vi "Set Defaults.vi"(8 "error in":errorcluster, 11 "VISA resource name":refnum<visa-resource-name>) -> (0 "error out":errorcluster, 3 "VISA resource name out":refnum<visa-resource-name>)   [LabVIEW 2019, in "Acopian.lvlib" / "Acopian.lvclass"]
uses:
  Library/Acopian.lvclass
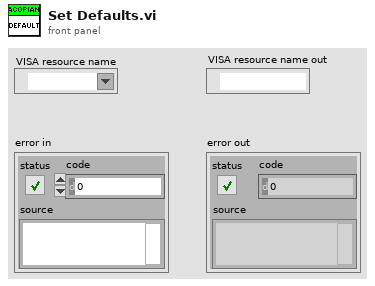
[diagram p1: front panel]
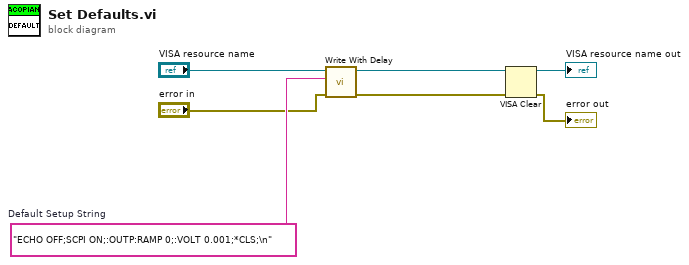
[diagram p0: block diagram]
diagram:
  w4 = "ECHO OFF;SCPI ON;:OUTP:RAMP 0;:VOLT 0.001;*CLS;\n"  # Default Setup String
  n1 = call "Write With Delay.vi"("error in"="error in", "write buffer"=w4, "VISA resource name"="VISA resource name") -> ("error out"=w1:errorcluster, "VISA resource name out"=w2:refnum<visa-resource-name>)  [unwired: 7 in]
  n2 = VISA Clear(VISA resource name=w2, error in (no error)=w1) -> (VISA resource name out=→"VISA resource name out":refnum<visa-resource-name>, error out=→"error out":errorcluster)
